vi "readconditional.vi"() -> ()   [LabVIEW 2014]
panel:
  out "output":string
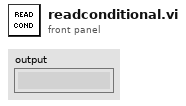
[diagram p1: front panel]
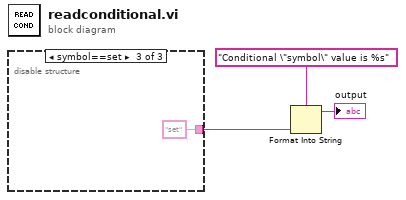
[diagram p0: block diagram]
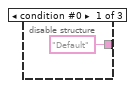
[diagram p2: hidden frame]
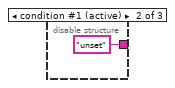
[diagram p3: hidden frame]
diagram:
  n1 = disable-structure shown="symbol==set" {
    disable-tunnel: ["Default" ("input 1") "unset" ("input 1") "set" ("input 1")] -> w1
    frame condition #0 {
    }
    frame condition #1 (active) {
    }
    frame condition #2 {
    }
  }
  n2 = Format Into String(format string="Conditional \"symbol\" value is %s", w1) -> (resulting string=→"output":string)  [unwired: 2 in, 1 out]
